vi "hse-application_ValidateConfigAndDataDirectories.vi"(8 "error in (no error)":errorcluster, 10 "Data Directory":path, 11 "Config Directory":path) -> (0 "error out":errorcluster, 2 "Data Directory DUP":path, 3 "Config Directory DUP":path)   [LabVIEW 2014, in "hse-application.lvclass"]
uses:
  hse-application.lvclass
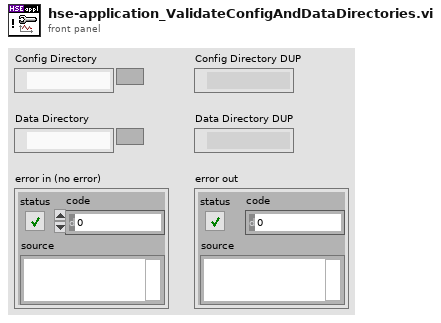
[diagram p1: front panel]
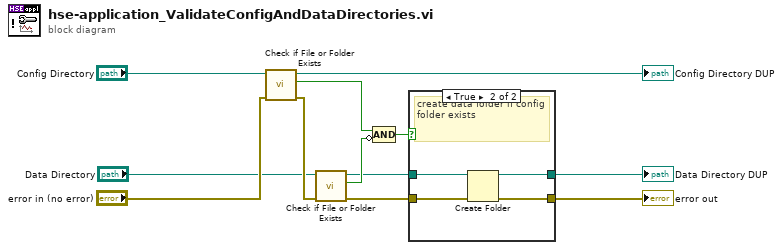
[diagram p0: block diagram]
diagram:
  n1 = call <vilib>:"Check if File or Folder Exists.vi"("error in (no error)"="error in (no error)", "path"="Config Directory") -> ("error out"=w11:errorcluster, "file or folder exists?"=w6:bool, "dup path"=→"Config Directory DUP":path)  [unwired: 7 in]
  n2 = call <vilib>:"Check if File or Folder Exists.vi"("error in (no error)"=w11, "path"="Data Directory") -> ("error out"=w4:errorcluster, "file or folder exists?"=w7:bool, "dup path"=w2:path)  [unwired: 7 in]
  n3 = Compound Arithmetic op=AND(w6, invert w7) -> (w8:bool)
  n4 = case shown="True" w8 {
    tunnel: w2 -> [w14 w18]
    tunnel: [w14 w17] -> w3
    tunnel: w4 -> [w13 w16]
    tunnel: [w13 w15] -> w5
    frame False {
    }
    frame True {
      # "create data folder if config folder exists"
      n5 = Create Folder(path (use dialog)=w18, error in=w16) -> (created path=w17:path, error out=w15:errorcluster)  [unwired: 1 in, 1 out]
    }
  }
  "error out" <- w5
  "Data Directory DUP" <- w3
